vi "Lookup Related Entities.vi"(6 "Relation":T1, 8 "error in (no error)":errorcluster, 9 "Primary ID":T3, 10 "Types":refnum<class "Type.lvclass">[](array[class]), 11 "Database in":refnum<class "SQLite.lvclass">) -> (0 "error out":errorcluster, 2 "Results":refnum<class "Result Row.lvclass">[](array[class]), 3 "Database out":refnum<class "SQLite.lvclass">)   [LabVIEW 2020, in "Conditum SQLite.lvlib" / "SQLite.lvclass"]
uses:
  SQLite.lvclass
  SQLite.lvclass/SQLite.ctl
  <vilib>/drjdpowell/SQLite Library/SQL Connection/Connection.lvclass
  <vilib>/drjdpowell/SQLite Library/SQL Statement/SQL Statement.lvclass
  <vilib>/IlluminatedG/IG Conditum Base/Conditum/Columns/Type/Type.lvclass
  <vilib>/IlluminatedG/IG Conditum Base/Conditum/Columns/Boolean/Boolean.lvclass
  <vilib>/IlluminatedG/IG Conditum Base/Conditum/Columns/Integer/Integer.lvclass
  <vilib>/IlluminatedG/IG Conditum Base/Conditum/Columns/ID/ID.lvclass
  <vilib>/IlluminatedG/IG Conditum Base/Conditum/Columns/Double/Double.lvclass
  <vilib>/IlluminatedG/IG Conditum Base/Conditum/Columns/Timestamp/Timestamp.lvclass
  <vilib>/IlluminatedG/IG Conditum Base/Conditum/Columns/String/String.lvclass
  <vilib>/IlluminatedG/IG Conditum Base/Conditum/Database Platform/Database Platform.lvclass
  C:/Program Files (x86)/National Instruments/LabVIEW 2020/vi.lib/IlluminatedG/IG Conditum Base/Conditum/Columns/Type/Type.lvclass
  C:/Program Files (x86)/National Instruments/LabVIEW 2020/vi.lib/IlluminatedG/IG Conditum Base/Conditum/Columns/Boolean/Boolean.lvclass
  C:/Program Files (x86)/National Instruments/LabVIEW 2020/vi.lib/IlluminatedG/IG Conditum Base/Conditum/Columns/Integer/Integer.lvclass
  C:/Program Files (x86)/National Instruments/LabVIEW 2020/vi.lib/IlluminatedG/IG Conditum Base/Conditum/Columns/ID/ID.lvclass
  C:/Program Files (x86)/National Instruments/LabVIEW 2020/vi.lib/IlluminatedG/IG Conditum Base/Conditum/Columns/Double/Double.lvclass
  C:/Program Files (x86)/National Instruments/LabVIEW 2020/vi.lib/IlluminatedG/IG Conditum Base/Conditum/Columns/Timestamp/Timestamp.lvclass
  C:/Program Files (x86)/National Instruments/LabVIEW 2020/vi.lib/IlluminatedG/IG Conditum Base/Conditum/Columns/String/String.lvclass
  C:/Program Files (x86)/National Instruments/LabVIEW 2020/vi.lib/IlluminatedG/IG Conditum Base/Conditum/Database Platform/Database Platform.lvclass
  C:/dev/lv20CE/lv-conditum-sqlite/Conditum SQLite/SQLite/SQLite.lvclass
  <vilib>/IlluminatedG/IG Conditum Base/Conditum/Entity ID.ctl
  <vilib>/IlluminatedG/IG Conditum Base/Conditum/Conditum.lvlib
  <vilib>/IlluminatedG/IG Conditum Base/Conditum/Relation Mapping.ctl
  <vilib>/IlluminatedG/IG Conditum Base/Conditum/Columns/Relation/Relation Info.ctl
  <vilib>/IlluminatedG/IG Conditum Base/Conditum/Result Row/Result Row.lvclass
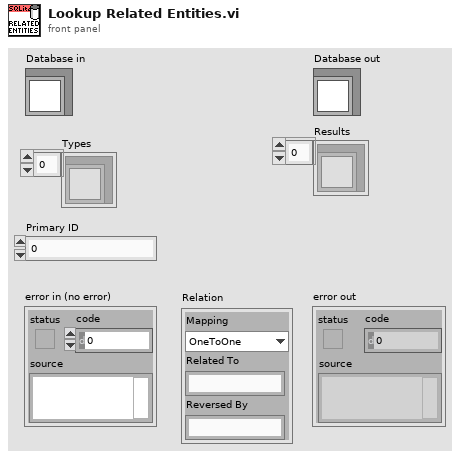
[diagram p1: front panel]
types:
  T1 = typedef "Conditum.lvlib/Relation Info.ctl" = cluster{"Mapping":T2, "Related To":string, "Reversed By":string}
  T2 = typedef "Conditum.lvlib/Relation Mapping.ctl" = enum16{"OneToOne", "OneToMany", "ManyToOne", "ManyToMany"}
  T3 = typedef "Conditum.lvlib/Entity ID.ctl" = i64
  T4 = typedef "Conditum.lvlib/Field Type.ctl" = enum16{"None", "ID", "Boolean", "Integer", "Double", "Timestamp", "String", "Text", "Entity"}
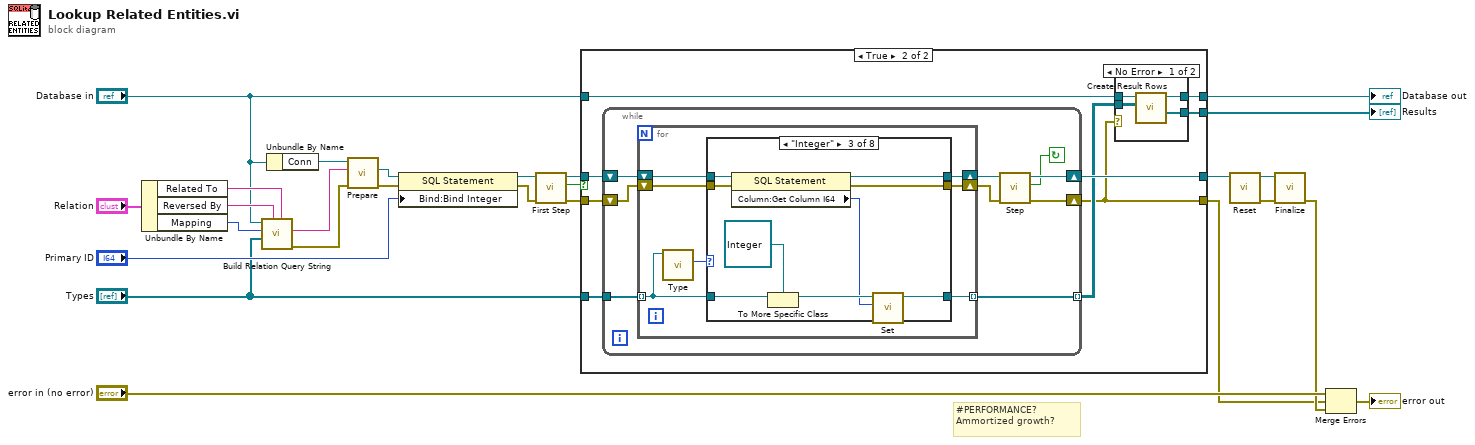
[diagram p0: block diagram]
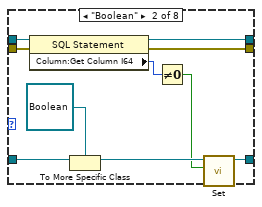
[diagram p5: hidden frame]
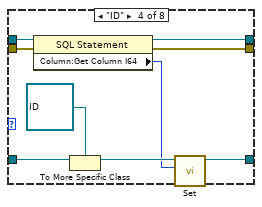
[diagram p6: hidden frame]
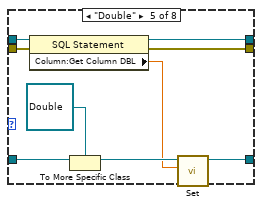
[diagram p7: hidden frame]
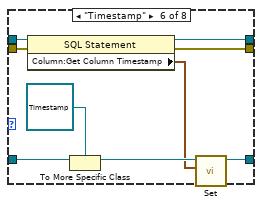
[diagram p8: hidden frame]
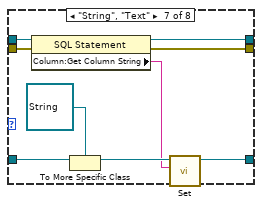
[diagram p9: hidden frame]
diagram:
  # "#PERFORMANCE?\nAmmortized growth?"
  n1 = Unbundle By Name("Relation") -> ("Related To"=w23:string, "Reversed By"=w24:string, "Mapping"=w25:T2)
  n2 = call "Build Relation Query String.vi"("Related To Table Name"=w23, "Reversed By Column Name"=w24, "Types"="Types", "From Mapping"=w25, "SQLite in"="Database in") -> ("error out"=w19:errorcluster, "Query String"=w21:string)  [unwired: 5 in]
  n3 = Unbundle By Name("Database in") -> ("Conn"=w22:refnum<class "Connection.lvclass">)
  n4 = call <vilib>:"Prepare.vi"("error in (no error)"=w19, "SQL"=w21, "SQLite Connection in"=w22) -> ("error out"=w20:errorcluster, "SQL Statement"=w18:refnum<class "SQL Statement.lvclass">)  [unwired: 4 in, 3 out]
  n5 = property class="SQL Statement"(reference=w18, error in=w20, "Bind:Bind Integer"="Primary ID") -> (reference out=w16:refnum<class "SQL Statement.lvclass">, error out=w15:errorcluster)
  n6 = call <vilib>:"First Step.vi"("error in (no error)"=w15, "SQL Statement in"=w16) -> ("error out"=w12:errorcluster, "Row returned"=w14:bool, "SQL Statement"=w13:refnum<class "SQL Statement.lvclass">)  [unwired: 7 in]
  n7 = case shown="True" w14 {
    tunnel: w13 -> [w29 w38]
    tunnel: w12 -> [w28 w37]
    tunnel: "Types" -> [_ w36]
    tunnel: [w29 w35] -> w8
    tunnel: "Database in" -> [w27 w34]
    tunnel: [w27 w33] -> w6
    tunnel: [w28 w31] -> w3
    tunnel: [_ w30] -> w1
    frame False {
    }
    frame True {
      n8 = while {
        shift-right: [w47] -> w35
        shift-left: w38 -> [w52]
        shift-right: [w46] -> w31
        shift-left: w37 -> [w50]
        tunnel: w36 -> [w51]
        tunnel: [w44] -> w32 mode=indexing
        stop <- w45 continue-if-true
        n9 = for {
          shift-right: [w55] -> w49
          shift-left: w52 -> [w59]
          tunnel: w51 -> [w56] mode=indexing
          tunnel: [w53] -> w44 mode=indexing
          shift-right: [w54] -> w48
          shift-left: w50 -> [w58]
          n10 = call <vilib>:"Type.vi"("Type in"=w56) -> ("Type"=w57:T4)  [unwired: 10 in]
          n11 = case shown="\"Integer\"" w57 {
            tunnel: w59 -> [w61 w69 w78 w87 w96 w105 w114 w118]
            tunnel: w58 -> [w60 w68 w77 w86 w95 w104 w113 w117]
            tunnel: w56 -> [_ w71 w80 w89 w98 w107 w116 _]
            tunnel: [w61 w67 w76 w85 w94 w103 w112 w118] -> w55
            tunnel: [w60 w66 w75 w84 w93 w102 w111 w117] -> w54
            tunnel: [_ w62 w72 w81 w90 w100 w108 _] -> w53
            frame "None", Default {
              # "#ERROR"
            }
            frame "Boolean" {
              n12 = property class="SQL Statement"(reference=w69, error in=w68) -> (reference out=w67:refnum<class "SQL Statement.lvclass">, error out=w66:errorcluster, "Column:Get Column I64"=w65:i64)
              n13 = To More Specific Class(target class=refnum<class "Boolean.lvclass"> refnum ("Conditum:Columns:Boolean.lvclass"), reference=w71) -> (specific class reference=w64:refnum<class "Boolean.lvclass">)  [unwired: 1 in, 1 out]
              n14 = Not Equal To 0?(x=w65) -> (x != 0?=w63:bool)
              n15 = call <vilib>:"Set.vi"("Value"=w63, "Boolean in"=w64) -> ("Boolean out"=w62:refnum<class "Boolean.lvclass">)  [unwired: 9 in]
            }
            frame "Integer" {
              n16 = property class="SQL Statement"(reference=w78, error in=w77) -> (reference out=w76:refnum<class "SQL Statement.lvclass">, error out=w75:errorcluster, "Column:Get Column I64"=w73:i64)
              n17 = To More Specific Class(target class=refnum<class "Integer.lvclass"> refnum ("Conditum:Columns:Integer.lvclass"), reference=w80) -> (specific class reference=w74:refnum<class "Integer.lvclass">)  [unwired: 1 in, 1 out]
              n18 = call <vilib>:"Set.vi"("Value"=w73, "Integer in"=w74) -> ("Integer out"=w72:refnum<class "Integer.lvclass">)  [unwired: 9 in]
            }
            frame "ID" {
              n19 = property class="SQL Statement"(reference=w87, error in=w86) -> (reference out=w85:refnum<class "SQL Statement.lvclass">, error out=w84:errorcluster, "Column:Get Column I64"=w82:i64)
              n20 = To More Specific Class(target class=refnum<class "ID.lvclass"> refnum ("Conditum:Columns:ID.lvclass"), reference=w89) -> (specific class reference=w83:refnum<class "ID.lvclass">)  [unwired: 1 in, 1 out]
              n21 = call <vilib>:"Set.vi"("Entity ID"=w82, "ID in"=w83) -> ("ID out"=w81:refnum<class "ID.lvclass">)  [unwired: 9 in]
            }
            frame "Double" {
              n22 = property class="SQL Statement"(reference=w96, error in=w95) -> (reference out=w94:refnum<class "SQL Statement.lvclass">, error out=w93:errorcluster, "Column:Get Column DBL"=w91:dbl)
              n23 = To More Specific Class(target class=refnum<class "Double.lvclass"> refnum ("Conditum:Columns:Double.lvclass"), reference=w98) -> (specific class reference=w92:refnum<class "Double.lvclass">)  [unwired: 1 in, 1 out]
              n24 = call <vilib>:"Set.vi"("Value"=w91, "Double in"=w92) -> ("Double out"=w90:refnum<class "Double.lvclass">)  [unwired: 9 in]
            }
            frame "Timestamp" {
              n25 = property class="SQL Statement"(reference=w105, error in=w104) -> (reference out=w103:refnum<class "SQL Statement.lvclass">, error out=w102:errorcluster, "Column:Get Column Timestamp"=w99:timestamp)
              n26 = To More Specific Class(target class=refnum<class "Timestamp.lvclass"> refnum ("Conditum:Columns:Timestamp.lvclass"), reference=w107) -> (specific class reference=w101:refnum<class "Timestamp.lvclass">)  [unwired: 1 in, 1 out]
              n27 = call <vilib>:"Set.vi"("Time Stamp"=w99, "DateTime in"=w101) -> ("DateTime out"=w100:refnum<class "Timestamp.lvclass">)  [unwired: 9 in]
            }
            frame "String", "Text" {
              n28 = property class="SQL Statement"(reference=w114, error in=w113) -> (reference out=w112:refnum<class "SQL Statement.lvclass">, error out=w111:errorcluster, "Column:Get Column String"=w109:string)
              n29 = To More Specific Class(target class=refnum<class "String.lvclass"> refnum ("Conditum:Columns:String.lvclass"), reference=w116) -> (specific class reference=w110:refnum<class "String.lvclass">)  [unwired: 1 in, 1 out]
              n30 = call <vilib>:"Set.vi"("Value"=w109, "String in"=w110) -> ("String out"=w108:refnum<class "String.lvclass">)  [unwired: 9 in]
            }
            frame "Entity" {
              # "#TODO\nRelation update"
            }
          }
        }
        n31 = call <vilib>:"Step.vi"("error in (no error)"=w48, "SQL Statement in"=w49) -> ("error out"=w46:errorcluster, "Row returned"=w45:bool, "SQL Statement"=w47:refnum<class "SQL Statement.lvclass">)  [unwired: 7 in]
      }
      n32 = case shown="No Error" w31 {
        tunnel: w34 -> [w42 w43]
        tunnel: [w41 w43] -> w33
        tunnel: w32 -> [w40 _]
        tunnel: [w39 _] -> w30
        frame No Error {
          n33 = call <vilib>:"Create Result Rows.vi"("Values"=w40, "Database in"=w42) -> ("Results"=w39:refnum<class "Result Row.lvclass">[], "Database out"=w41:refnum<class "SQLite.lvclass">)  [unwired: 8 in]
        }
        frame Error {
        }
      }
    }
  }
  "Database out" <- w6
  "Results" <- w1
  n34 = call <vilib>:"Reset.vi"("SQL Statement in"=w8) -> ("error out"=w9:errorcluster, "SQL Statement"=w10:refnum<class "SQL Statement.lvclass">)  [unwired: 9 in]
  n35 = call <vilib>:"Finalize.vi"("error in (no error)"=w9, "SQL Statement in"=w10) -> ("error out"=w4:errorcluster)  [unwired: 9 in]
  n36 = Merge Errors("error in (no error)", w3, w4) -> (→"error out":errorcluster)
